vi "Uncertainty.vi"(0 "Number":dbl, 1 "Slope":dbl=90.0) -> (2 "Incertezza\nAttendibile":bool=TRUE, 3 "Incertezza\nin uscita":dbl=0.3741657386773941, 4 "Incertezza\nComposta":dbl=101.02474944289642)   [LabVIEW 2021]
uses:
  <vilib>/Analysis/NI_AALBase.lvlib
panel:
  out "Calcolo Dinamico\nIncertezza":dbl=nan
  out "Deviazione standard":dbl=-0.0 format="%0.2f"
  out "Elapsed Time (s)":dbl=2.0014543533325195
  in  "stop":bool
  out "Dimensione\narray":i32
  out "Build\nArray":dbl[](array[numeric])
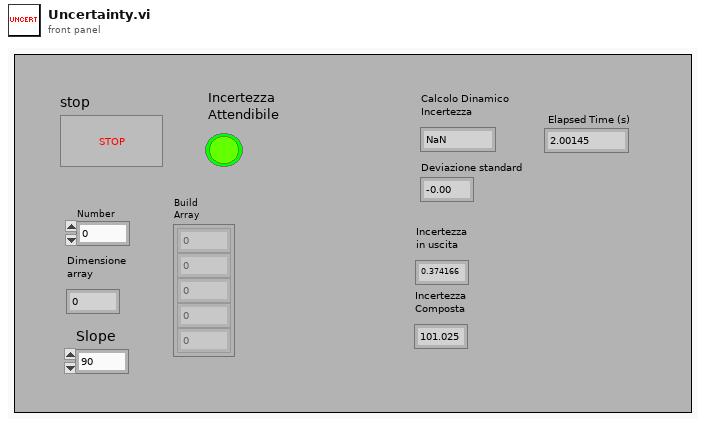
[diagram p1: front panel]
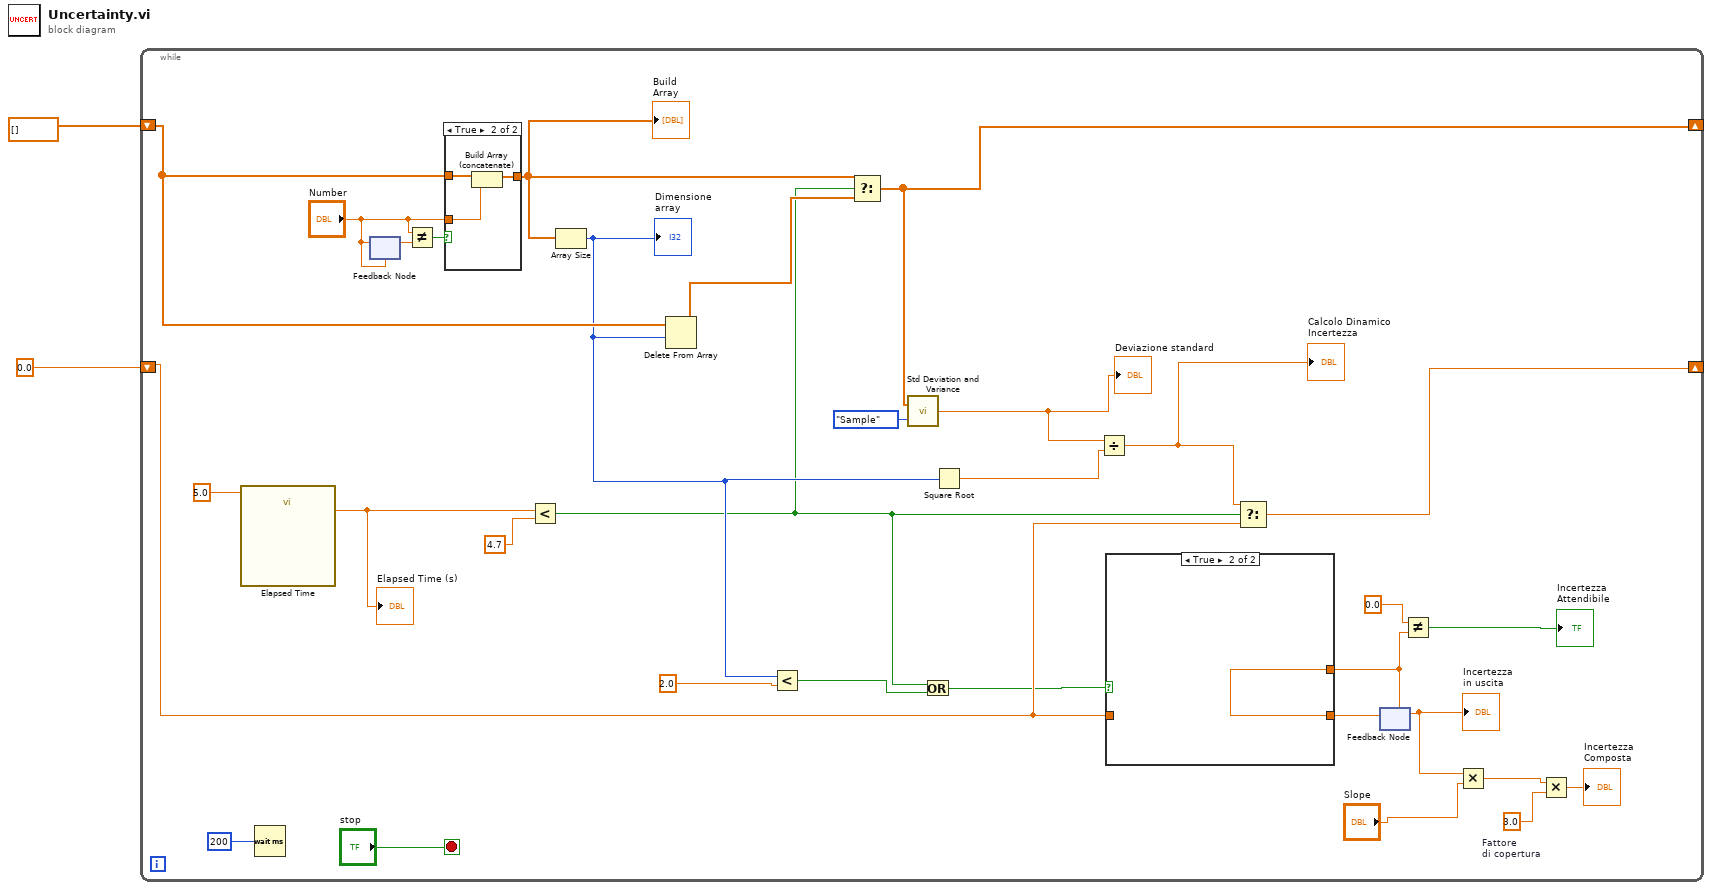
[diagram p0: block diagram]
diagram:
  n1 = while {
    shift-right: [w24] -> _
    shift-left: dbl[] [] -> [w28]
    shift-right: [w20] -> _
    shift-left: 0.0 -> [w16]
    stop <- "stop" stop-if-true
    w4 = 3.0  # Fattore di copertura
    n2 = call "Elapsed Time"("Time Target (s)"=5.0) -> ("Elapsed Time (s)"=w21:dbl)  [unwired: 11 in, 7 out]
    "Elapsed Time (s)" <- w21
    n3 = Wait (ms)(milliseconds to wait=u32 200) -> ()  [unwired: 1 out]
    n4 = feedback-in #1("Number") -> ()
    n5 = feedback #1("Number") -> (w32:dbl)
    n6 = Not Equal?(x="Number", y=w32) -> (x != y?=w30:bool)
    n7 = case shown="True" w30 {
      tunnel: "Number" -> [_ w39]
      tunnel: [w36 w38] -> w27
      tunnel: w28 -> [w36 w37]
      frame False {
      }
      frame True {
        n8 = Build Array (concatenate)(w37, w39) -> (w38:dbl[])
      }
    }
    "Build\nArray" <- w27
    n9 = Less?(x=w21, y=4.7) -> (x < y?=w10:bool)
    n10 = Array Size(array=w27) -> (size(s)=w12:i32)
    "Dimensione\narray" <- w12
    n11 = Delete From Array(array=w28, length=w12) -> (array with subset deleted=w26:dbl[])  [unwired: 1 in, 1 out]
    n12 = Less?(x=w12, y=2.0) -> (x < y?=w11:bool)
    n13 = Select(t=w27, s=w10, f=w26) -> (s? t:f=w24:dbl[])
    n14 = call <vilib>:"Std Deviation and Variance.vi"("X"=w24, "Weighting (Sample)"=enum16{"Sample", "Population"}."Sample") -> ("standard deviation"=w23:dbl)  [unwired: 2 out]
    "Deviazione standard" <- w23
    n15 = Or(x=w10, y=w11) -> (x .or. y?=w9:bool)
    n16 = Square Root(x=w12) -> (sqrt(x)=w25:dbl)
    n17 = Divide(x=w23, y=w25) -> (x/y=w18:dbl)
    "Calcolo Dinamico\nIncertezza" <- w18
    n18 = Select(t=w18, s=w10, f=w16) -> (s? t:f=w20:dbl)
    n19 = feedback #2() -> (w7:dbl)  [unwired: 1 in]
    "Incertezza\nin uscita" <- w7
    n20 = case shown="True" w9 {
      tunnel: w16 -> [w34 _]
      tunnel: [w34 w35] -> w19
      tunnel: w7 -> [_ w35]
      frame False {
      }
      frame True {
      }
    }
    n21 = feedback-in #2(w19) -> ()
    n22 = Not Equal?(x=0.0 ("y"), y=w7) -> (x != y?=→"Incertezza\nAttendibile":bool)
    n23 = Multiply(x=w7, y="Slope") -> (x*y=w5:dbl)
    n24 = Multiply(x=w5, y=w4) -> (x*y=→"Incertezza\nComposta":dbl)
  }
